vi "TagMetadataToImage.vi"(8 "error in (no error)":errorcluster, 10 "Image In":T1, 11 "StepMotorController in":refnum<class "StepMotorController.lvclass">) -> (0 "error out":errorcluster, 2 "Image Out":T1, 3 "StepMotorController out":refnum<class "StepMotorController.lvclass">)   [LabVIEW 2020, in "StepMotorController.lvlib" / "StepMotorController.lvclass"]
uses:
  StepMotorController.lvclass
  <vilib>/vision/Image Controls.llb/IMAQ Image.ctl
  StepMotorController.lvclass/StepMotorController.ctl
  Model/Hardware Abstraction Layer/Component/GenericActor/GenericActor/GenericController.lvclass
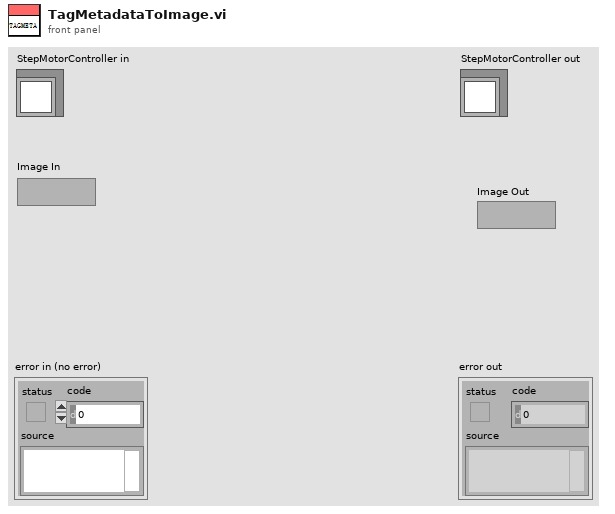
[diagram p1: front panel]
types:
  T1 = typedef "IMAQ Image.ctl" = refnum<image>
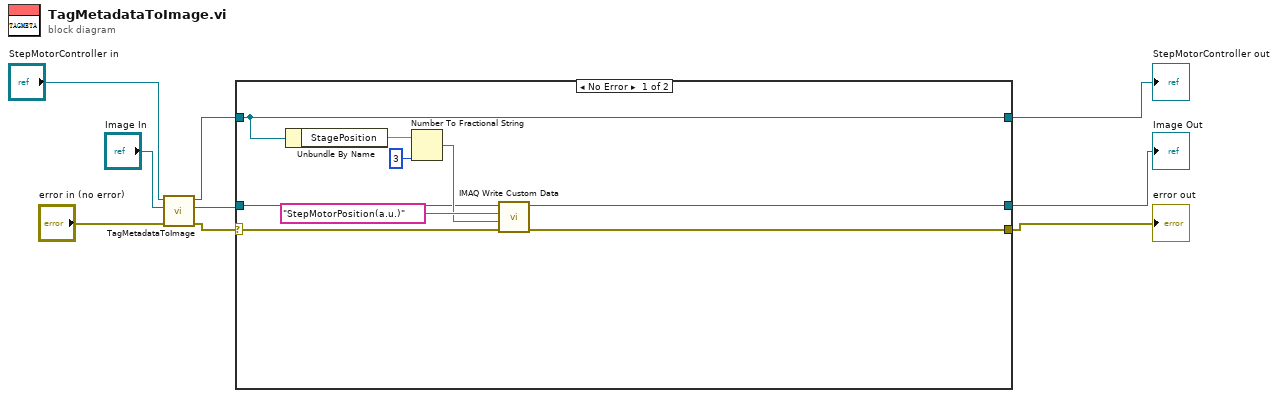
[diagram p0: block diagram]
diagram:
  n1 = call-parent "TagMetadataToImage.vi"("error in (no error)"="error in (no error)", "Image In"="Image In", "GenericController in"="StepMotorController in") -> ("error out"=w6:errorcluster, "Image Out"=w5:T1, "GenericController out"=w4:refnum<class "StepMotorController.lvclass">)  [unwired: 6 in]
  n2 = case shown="No Error" w6 {
    selector: w6 -> [w17 w21]
    tunnel: [w16 w21] -> w1
    tunnel: w5 -> [w13 w20]
    tunnel: [w12 w20] -> w2
    tunnel: [w18 w19] -> w3
    tunnel: w4 -> [w18 w19]
    frame No Error {
      n3 = Unbundle By Name(w18) -> ("StagePosition"=w10:dbl)
      n4 = Number To Fractional String(number=w10, precision (6)=i16 3 ("width (-)")) -> (F-format string=w14:string)  [unwired: 2 in]
      n5 = call "IMAQ Write Custom Data"("error in (no error)"=w17, "Custom Data In"=w14, "Key"="StepMotorPosition(a.u.)", "Image"=w13) -> ("error out"=w16:errorcluster, "Image Out"=w12:T1)  [unwired: 6 in]
    }
    frame Error {
    }
  }
  "error out" <- w1
  "StepMotorController out" <- w3
  "Image Out" <- w2
